vi "__Build Cloud path.vi"(6 "Folder?":bool=TRUE, 10 "New Path element":string, 11 "Current Cloud path":string) -> (3 "New Cloud path":string)   [LabVIEW 2011]
doc: "This VI appends a new element to the current cloud path."
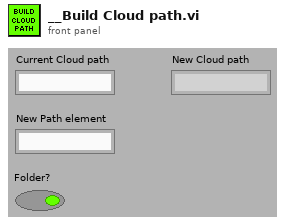
[diagram p1: front panel]
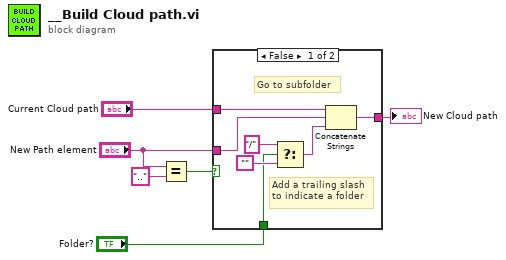
[diagram p0: block diagram]
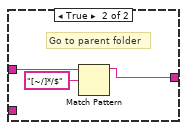
[diagram p2: hidden frame]
diagram:
  n1 = Equal?(x="New Path element", y="..") -> (x = y?=w5:bool)
  n2 = case shown="False" w5 {
    tunnel: "New Path element" -> [w12 _]
    tunnel: "Current Cloud path" -> [w13 w16]
    tunnel: [w11 w14] -> w2
    tunnel: "Folder?" -> [w9 _]
    frame False {
      # "Add a trailing slash\nto indicate a folder"
      # "Go to subfolder"
      n3 = Select(t="/", s=w9, f="" ("string")) -> (s? t:f=w7:string)
      n4 = Concatenate Strings(w13, w12, w7) -> (w11:string)
    }
    frame True {
      # "Go to parent folder"
      n5 = Match Pattern(string=w16, regular expression="[~/]*/$") -> (before substring=w14:string)  [unwired: 1 in, 3 out]
    }
  }
  "New Cloud path" <- w2
